vi "Get Pulse Time.vi"(0 "Arduino Resource":T1={"VISA resource"="", "Board Type"=enum."Uno", "Connection Type"=enum."USB / Serial", "Bytes Per Packet (15)"=15}, 5 "Trigger Pin":u8, 7 "Signal Pin":u8, 11 "error in (no error)":errorcluster, 13 "Trigger Length (us)":u8=5) -> (4 "Arduino Resource":T1={"VISA resource"="", "Board Type"=enum."Uno", "Connection Type"=enum."USB / Serial", "Bytes Per Packet (15)"=15}, 8 "Pulse Time (us)":u32, 15 "error out":errorcluster)   [LabVIEW 2012, in "LIFA Ultrasonic Distance.lvlib"]
doc: "Sends a trigger pulse and returns the width of the returned pulse in microseconds.\nCustom firmware is required to run this VI."
uses:
  LIFA Ultrasonic Distance.lvlib
  <vilib>/LabVIEW Interface for Arduino/LabVIEW Interface for Arduino.lvlib
  <vilib>/LabVIEW Interface for Arduino/Type Defs/Board Type.ctl
  <vilib>/LabVIEW Interface for Arduino/Type Defs/Arduino Resource.ctl
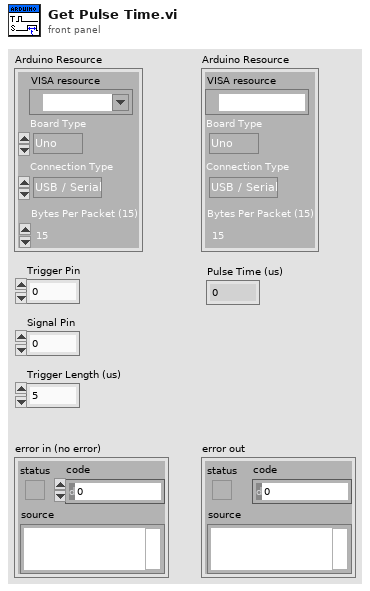
[diagram p1: front panel]
types:
  T1 = typedef "LabVIEW Interface for Arduino.lvlib/Arduino Resource.ctl" = cluster{"VISA resource":refnum<visa-resource-name>, "Board Type":T2, "Connection Type":enum8{"USB / Serial"}, "Bytes Per Packet (15)":u8}
  T2 = typedef "LabVIEW Interface for Arduino.lvlib/Board Type.ctl" = enum16{"Uno", "Dimuelanove w/Atmega 328", "Mega 2560"}
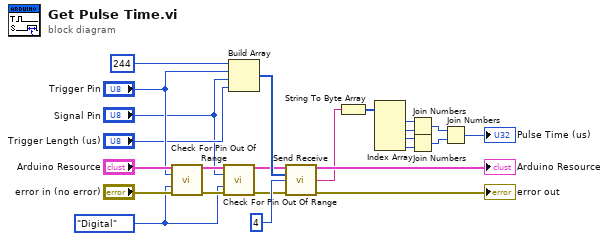
[diagram p0: block diagram]
diagram:
  w5 = enum16{"Analog", "Digital"}."Digital" ("Pin Type")
  n1 = call <vilib>:"Check For Pin Out Of Range.vi"("Arduino Resource"="Arduino Resource", "User Pin Number"="Trigger Pin", "Pin Type"=w5, "error in"="error in (no error)") -> ("Arduino Resource"=w7:T1, "error out"=w6:errorcluster)  [unwired: 10 in]
  n2 = call <vilib>:"Check For Pin Out Of Range.vi"("Arduino Resource"=w7, "User Pin Number"="Signal Pin", "Pin Type"=w5, "error in"=w6) -> ("Arduino Resource"=w3:T1, "error out"=w2:errorcluster)  [unwired: 10 in]
  n3 = Build Array(u8 244, "Trigger Pin", "Signal Pin", "Trigger Length (us)") -> (w22:u8[])
  n4 = call <vilib>:"Send Receive.vi"("Arduino Resource"=w3, "Data"=w22, "Bytes To Read (0)"=u8 4, "error in"=w2) -> ("Arduino Resource"=→"Arduino Resource":T1, "Read Buffer"=w19:string, "error out"=→"error out":errorcluster)  [unwired: 9 in]
  n5 = String To Byte Array(string=w19) -> (unsigned byte array=w18:u8[])
  n6 = Index Array(array=w18) -> (element #1=w16:u8, element #2=w17:u8, element #3=w15:u8, element #4=w14:u8)  [unwired: 4 in]
  n7 = Join Numbers(hi=w16, lo=w17) -> ((hi.lo)=w12:u16)
  n8 = Join Numbers(hi=w15, lo=w14) -> ((hi.lo)=w13:u16)
  n9 = Join Numbers(hi=w12, lo=w13) -> ((hi.lo)=→"Pulse Time (us)":u32)
